vi "SVXMPL_Signal Generation (no HW).vi"(4 "noise amplitude":dbl=0.01 format="%.2f", 5 "pulse":T1={"square frequency"=20.0, "duty cycle (%)"=50.0} {"duty cycle (%)" format="%.2f"; "square frequency" format="%.2f"}, 6 "add noise (T)":bool=TRUE, 7 "pulsed (F)":bool, 8 "error in (no error)":errorcluster, 9 "window":T3(ring), 10 "df (dual tone)":dbl=100.0 format="%.2f", 11 "signal settings":T2={"signal type"=enum."Sine wave", "frequency"=1000.0, "amplitude"=1.0, "sampling info"={"sampling frequency"=51200.0, "#s"=4096.0}} {"sampling info"."#s" format="%.2f"; "sampling info"."sampling frequency" format="%.2p"; "amplitude" format="%.2f"; "frequency" format="%.2f"}) -> (0 "error out":errorcluster, 3 "signal out":waveform(dbl)={"t0"=timestamp(0 s since 1904-01-01), "dt"=4.5351473922902495e-05, "Y"=array[22050 elements]})   [LabVIEW 2017]
uses:
  <vilib>/measure/macond.llb/Scaled Window for 1 Chan.vi
  <vilib>/addons/_NISVFA/_Generation/SoundVib_Generation.lvlib
  <vilib>/measure/NI_MABase.lvlib
  <vilib>/Analysis/NI_AALBase.lvlib
  <vilib>/measure/NI_MAPro.lvlib
panel:
  out "Waveform Graph":waveform(dbl)(graph)={"t0"=timestamp(0 s since 1904-01-01), "dt"=4.5351473922902495e-05, "Y"=array[22050 elements]}
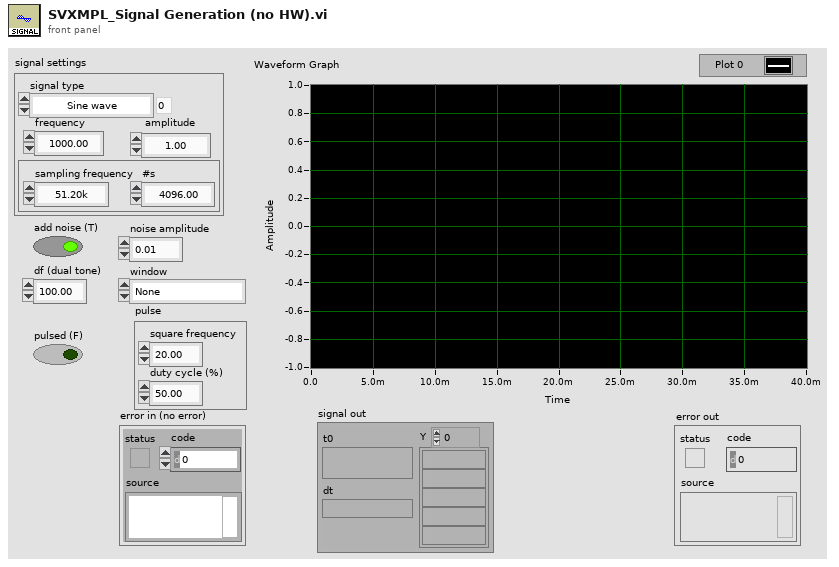
[diagram p1: front panel]
types:
  T1 = cluster{"square frequency":dbl, "duty cycle (%)":dbl}
  T2 = cluster{"signal type":enum16{"Sine wave", "Square wave", "Triangle wave", "Sawtooth wave", "Chirp", "Uniform white noise", "Gaussian white noise", "Pink noise", "PRN", "Dual tone"}, "frequency":dbl, "amplitude":dbl, "sampling info":cluster{"sampling frequency":dbl, "#s":dbl}}
  T3 = enum16{"None ", "Hanning", "Hamming", "Blackman-Harris", "Exact Blackman", "Blackman", "Flat Top", "4 Term B-Harris ", "7 Term B-Harris", "Low Sidelobe"}
  T4 = enum16{"Sine wave", "Square wave", "Triangle wave", "Sawtooth wave", "Chirp", "Uniform white noise", "Gaussian white noise", "Pink noise", "PRN", "Dual tone"}
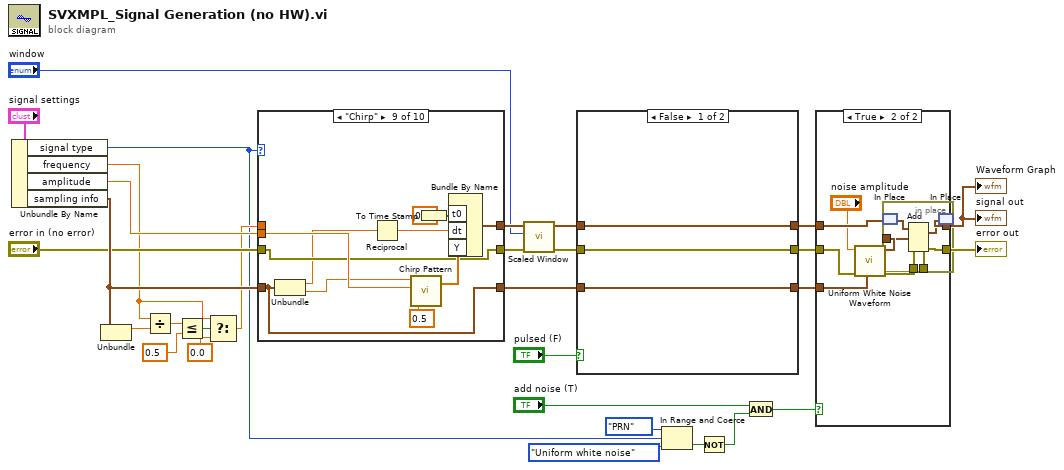
[diagram p0: block diagram]
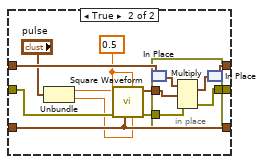
[diagram p2: hidden frame]
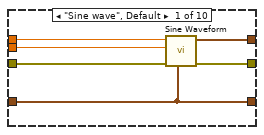
[diagram p4: hidden frame]
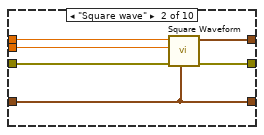
[diagram p5: hidden frame]
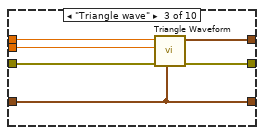
[diagram p6: hidden frame]
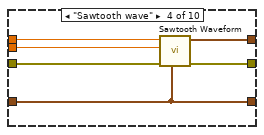
[diagram p7: hidden frame]
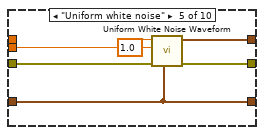
[diagram p8: hidden frame]
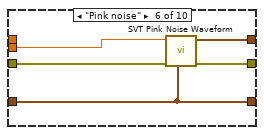
[diagram p9: hidden frame]
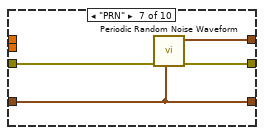
[diagram p10: hidden frame]
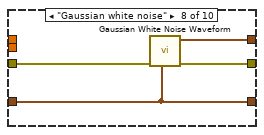
[diagram p11: hidden frame]
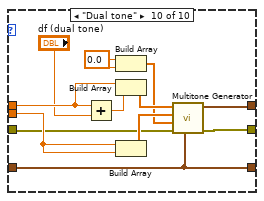
[diagram p12: hidden frame]
diagram:
  n1 = Unbundle By Name("signal settings") -> ("signal type"=w5:T4, "frequency"=w10:dbl, "amplitude"=w17:dbl, "sampling info"=w16:cluster{"sampling frequency":dbl, "#s":dbl})
  n2 = Unbundle(w16) -> ("sampling frequency"=w14:dbl)  [unwired: 1 out]
  n3 = Divide(x=w10, y=w14) -> (x/y=w13:dbl)
  n4 = Less Or Equal?(x=w13, y=0.5) -> (x <= y?=w11:bool)
  n5 = Select(t=w10, s=w11, f=0.0) -> (s? t:f=w9:dbl)
  n6 = case shown="\"Chirp\"" w5 {
    tunnel: w17 -> [w35 w41 w47 w53 w60 w64 _ _ w83 w90]
    tunnel: w16 -> [w32 w38 w44 w50 w57 w62 w67 w71 w84 w86]
    tunnel: w9 -> [w36 w42 w48 w54 _ _ _ _ _ w95]
    tunnel: [w34 w40 w46 w52 w59 w65 w69 w72 w82 w87] -> w28
    tunnel: [w33 w39 w45 w51 w58 w63 w68 w73 w77 w96] -> w27
    tunnel: [w32 w38 w44 w50 w57 w62 w67 w71 w84 w86] -> w23
    tunnel: "error in (no error)" -> [w31 w37 w43 w49 w56 w61 w66 w70 w77 w85]
    frame "Sine wave", Default {
      n7 = call <vilib>:"Sine Waveform.vi"("sampling info"=w32, "error in (no error)"=w31, "amplitude"=w35, "frequency"=w36) -> ("error out"=w33:errorcluster, "signal out"=w34:waveform(dbl))  [unwired: 6 in]
    }
    frame "Square wave" {
      n8 = call <vilib>:"Square Waveform.vi"("sampling info"=w38, "error in (no error)"=w37, "amplitude"=w41, "frequency"=w42) -> ("error out"=w39:errorcluster, "signal out"=w40:waveform(dbl))  [unwired: 6 in]
    }
    frame "Triangle wave" {
      n9 = call <vilib>:"Triangle Waveform.vi"("sampling info"=w44, "error in (no error)"=w43, "amplitude"=w47, "frequency"=w48) -> ("error out"=w45:errorcluster, "signal out"=w46:waveform(dbl))  [unwired: 6 in]
    }
    frame "Sawtooth wave" {
      n10 = call <vilib>:"Sawtooth Waveform.vi"("sampling info"=w50, "error in (no error)"=w49, "amplitude"=w53, "frequency"=w54) -> ("error out"=w51:errorcluster, "signal out"=w52:waveform(dbl))  [unwired: 6 in]
    }
    frame "Uniform white noise" {
      n11 = call <vilib>:"Uniform White Noise Waveform.vi"("sampling info"=w57, "error in (no error)"=w56, "seed"=1.0, "amplitude"=w60) -> ("error out"=w58:errorcluster, "signal out"=w59:waveform(dbl))  [unwired: 6 in]
    }
    frame "Pink noise" {
      n12 = call <vilib>:"SVT Pink Noise Waveform.vi"("sampling info"=w62, "error in (no error)"=w61, "amplitude"=w64) -> ("error out"=w63:errorcluster, "pink noise signal"=w65:waveform(dbl))  [unwired: 7 in]
    }
    frame "PRN" {
      n13 = call <vilib>:"Periodic Random Noise Waveform.vi"("sampling info"=w67, "error in (no error)"=w66) -> ("error out"=w68:errorcluster, "signal out"=w69:waveform(dbl))  [unwired: 8 in]
    }
    frame "Gaussian white noise" {
      n14 = call <vilib>:"Gaussian White Noise Waveform.vi"("sampling info"=w71, "error in (no error)"=w70) -> ("error out"=w73:errorcluster, "signal out"=w72:waveform(dbl))  [unwired: 8 in]
    }
    frame "Chirp" {
      n15 = Unbundle(w84) -> ("sampling frequency"=w75:dbl, "#s"=w76:dbl)
      n16 = Reciprocal(x=w75) -> (1/x=w79:dbl)
      n17 = call <vilib>:"Chirp Pattern.vi"("f2"=0.5, "amplitude"=w83, "samples"=w76) -> ("Chirp Pattern"=w81:dbl[])  [unwired: 1 in, 1 out]
      n18 = To Time Stamp(1:0.0 ("t0")) -> (0:w74:timestamp)
      n19 = Bundle By Name("t0"=w74, "dt"=w79, "Y"=w81) -> (w82:waveform(dbl))  [unwired: 1 in]
    }
    frame "Dual tone" {
      w89 = 0.0 ("Input Element")
      n20 = Add(x=w95, y="df (dual tone)") -> (x+y=w94:dbl)
      n21 = Build Array(w89, w89) -> (w88:dbl[])
      n22 = Build Array(w95, w94) -> (w93:dbl[])
      n23 = Build Array(w90, w90) -> (w91:dbl[])
      n24 = call <vilib>:"Multitone Generator.vi"("sampling info"=w86, "error in (no error)"=w85, "tone phases"=w88, "tone amplitudes"=w91, "tone frequencies"=w93) -> ("error out"=w96:errorcluster, "signal out"=w87:waveform(dbl))  [unwired: 3 in, 2 out]
    }
  }
  n25 = call-poly <vilib>:"Scaled Window.vi"("error in (no error)"=w27, "window"="window", "signal in"=w28) -> ("error out"=w24:errorcluster, "signal out"=w25:waveform(dbl))  [unwired: 6 in, 1 out]
  n26 = case shown="False" "pulsed (F)" {
    tunnel: w25 -> [w99 w110]
    tunnel: w24 -> [w98 w107]
    tunnel: w23 -> [w97 w103]
    tunnel: [w98 w106] -> w22
    tunnel: [w99 w105] -> w21
    tunnel: [w97 w103] -> w20
    frame False {
    }
    frame True {
      w104 = 0.5 ("amplitude")
      n27 = Unbundle("pulse") -> ("square frequency"=w101:dbl, "duty cycle (%)"=w100:dbl)
      n28 = call <vilib>:"Square Waveform.vi"("duty cycle (%)"=w100, "offset"=w104, "sampling info"=w103, "error in (no error)"=w107, "amplitude"=w104, "frequency"=w101) -> ("error out"=w108:errorcluster, "signal out"=w109:waveform(dbl))  [unwired: 4 in]
      n29 = in-place {
        in-place-border: w109 -> [w114]
        in-place-border: w108 -> [w113]
        in-place-border: [w112] -> w106
        n30 = in-place-match #1(w110) -> (w115:waveform(dbl))
        n31 = Multiply(1:w114, 2:w115, 4:w113) -> (0:w111:waveform(dbl), 3:w112:errorcluster)
        n32 = in-place-match #1(w111) -> (w105:waveform(dbl))
      }
    }
  }
  n33 = In Range and Coerce(upper limit=T4."PRN", x=w5, lower limit=T4."Uniform white noise") -> (In Range?=w6:bool)  [unwired: 1 out]
  n34 = Not(x=w6) -> (.not. x?=w1:bool)
  n35 = And(x="add noise (T)", y=w1) -> (x .and. y?=w7:bool)
  n36 = case shown="True" w7 {
    tunnel: w20 -> [_ w125]
    tunnel: w21 -> [w117 w124]
    tunnel: [w116 w122] -> w30
    tunnel: [w117 w121] -> w29
    tunnel: w22 -> [w116 w118]
    frame False {
    }
    frame True {
      n37 = call <vilib>:"Uniform White Noise Waveform.vi"("sampling info"=w125, "error in (no error)"=w118, "amplitude"="noise amplitude") -> ("error out"=w123:errorcluster, "signal out"=w120:waveform(dbl))  [unwired: 7 in]
      n38 = in-place {
        in-place-border: w123 -> [w129]
        in-place-border: [w128] -> w122
        in-place-border: w120 -> [w126]
        n39 = in-place-match #2(w124) -> (w130:waveform(dbl))
        n40 = Add(1:w126, 2:w130, 4:w129) -> (0:w127:waveform(dbl), 3:w128:errorcluster)
        n41 = in-place-match #2(w127) -> (w121:waveform(dbl))
      }
    }
  }
  "signal out" <- w29
  "error out" <- w30
  "Waveform Graph" <- w29
